vi "DAQ_FDV Meas Configure and Measure.vi"(0 "DAQmx Task In":refnum<k21>, 2 "Execution Settings":T1, 5 "Range and Terminal Settings":T6={"Global Settings"={"Min Range (V)"=-10.0, "Max Range (V)"=10.0, "Terminal Configuration"=10083}, "Specific Channel Settings"=[]} {"Specific Channel Settings"."Terminal Configuration" items=[""=0, "RSE"=10083, "NRSE"=10078, "Differential"=10106, "Pseudodifferential"=12529]; "Specific Channel Settings"."Max Range" format="%.2p"; "Specific Channel Settings"."Min Range" format="%.2p"; "Global Settings"."Terminal Configuration" items=["RSE"=10083, "NRSE"=10078, "Differential"=10106, "Pseudodifferential"=12529]; "Global Settings"."Max Range (V)" format="%.2p"; "Global Settings"."Min Range (V)" format="%.2p"}, 7 "Timing and Trigger Settings":T3={"Timing Settings"={"Sample Clock Source"="OnboardClock", "Sample Rate (Hz)"=10000.0, "Number of Samples"=1000, "Sample Timing Engine"=enum."Auto"}, "Trigger Settings"={"Trigger Type"=enum."No Trigger", "Digital Start Trigger Source"="", "Digital Start Trigger Edge"=10280}} {"Trigger Settings"."Digital Start Trigger Edge" items=["Rising"=10280, "Falling"=10171]; "Timing Settings"."Sample Rate (Hz)" format="%.2p"}, 11 "error in":errorcluster) -> (4 "DAQmx Task Out":refnum<k21>, 6 "Voltage Waveforms":waveform(dbl)[](graph), 8 "Frequency Domain Measurements":T8 {"Detected Tones"."Amplitudes (V)" format="%.2p"; "Detected Tones"."Frequencies (Hz)" format="%.2p"}, 10 "Acquisition Time (s)":dbl caption="Acq. Time Period (s)" format="%.2p", 15 "error out":errorcluster)   [LabVIEW 2021, in "DAQ_Frequency Domain Measurement.lvlib"]
doc: "Configure, initiate and fetch Frequency domain measurements from the channels configured."
uses:
  DAQ_Frequency Domain Measurement.lvlib
  Typedefs/Timing & Trigger Settings.ctl
  Typedefs/Timing Settings.ctl
  Signal Voltage Generation/Typedefs/Trigger Settings.ctl
  Typedefs/Range and Terminal Settings.ctl
  Typedefs/Specific Channel Settings.ctl
  Typedefs/FD Measurements.ctl
  Typedefs/Detected Tones.ctl
  Typedefs/Execution Settings.ctl
  Common/Typedefs/Execution Options - Measure.ctl
  <vilib>/DAQmx/read.llb/DAQmx Read (Analog 1D Wfm NChan NSamp).vi
  <vilib>/DAQmx/configure/timing.llb/DAQmx Timing (Sample Clock).vi
  <vilib>/DAQmx/configure/trigger.llb/DAQmx Start Trigger (Digital Edge).vi
  <vilib>/DAQmx/miscellaneous.llb/DAQmx Fill In Error Info.vi
  <resource>/objmgr/daqmx.rc
  Signal Voltage Generation/DAQ_Signal Voltage Generation.lvlib
panel:
  # "Inputs"
  # "Outputs"
  # "Min \nRange (V)"
  # "Max \nRange (V)"
  # "Terminal Configuration"
  # "Physical Channel Name"
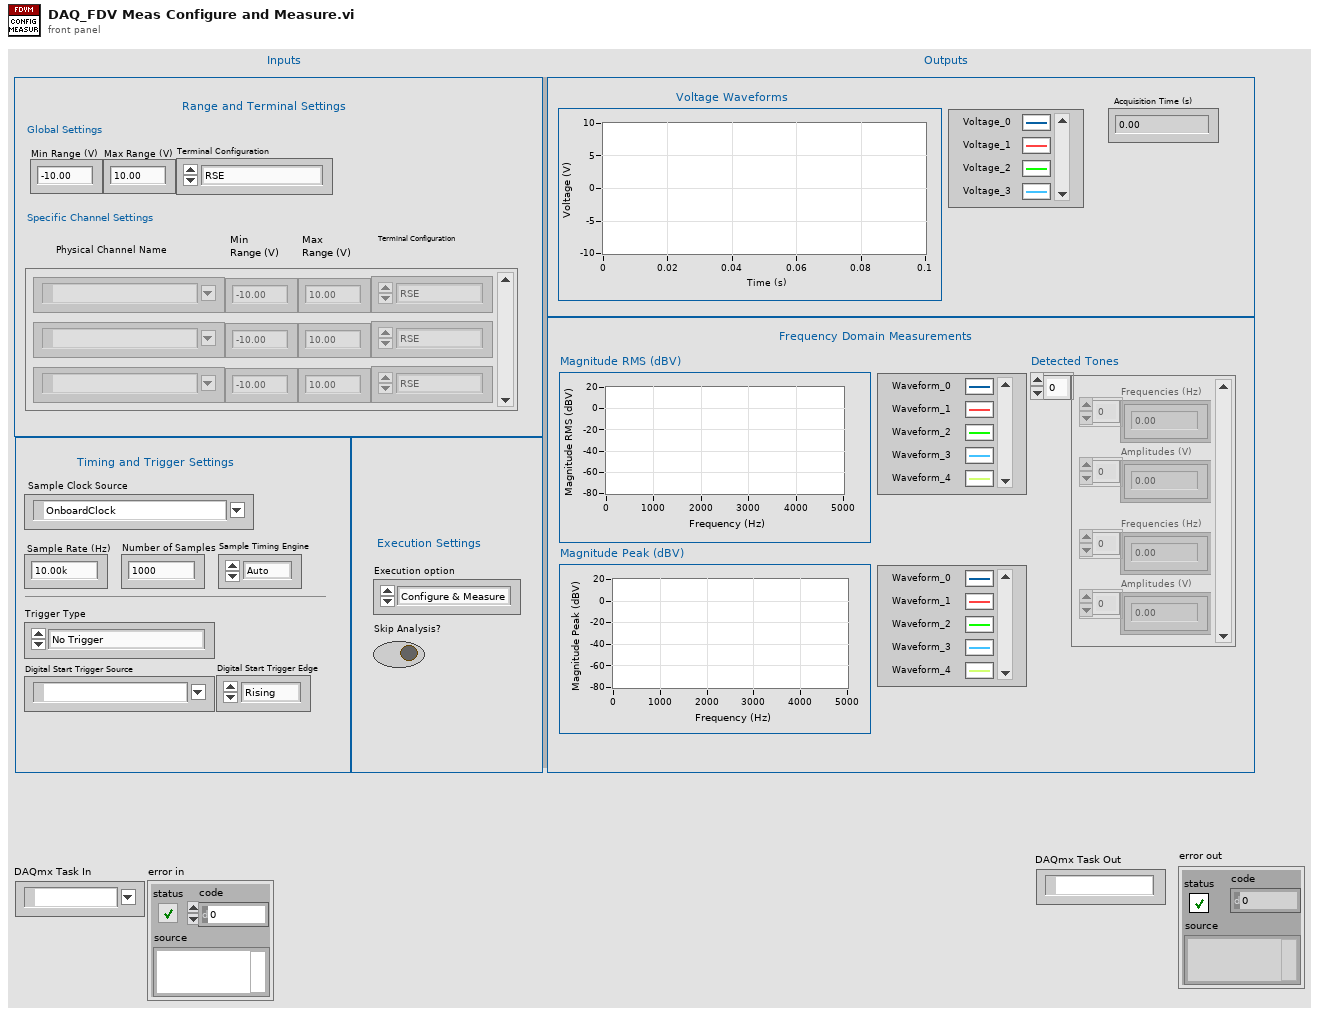
[diagram p1: front panel]
types:
  T1 = typedef "DAQ_Frequency Domain Measurement.lvlib/Execution Settings.ctl" = cluster{"Execution option":T2, "Skip Analysis?":bool}
  T2 = typedef "Execution Options - Measure.ctl" = enum16{"Configure & Measure", "Configure only", "Measure only"}
  T3 = typedef "DAQ_Frequency Domain Measurement.lvlib/Timing & Trigger Settings.ctl" = cluster{"Timing Settings":T4, "Trigger Settings":T5}
  T4 = typedef "DAQ_Frequency Domain Measurement.lvlib/Timing Settings.ctl" = cluster{"Sample Clock Source":tag, "Sample Rate (Hz)":dbl, "Number of Samples":i32, "Sample Timing Engine":enum16{"te0", "te1", "ai", "Auto"}}
  T5 = typedef "DAQ_Signal Voltage Generation.lvlib/Trigger Settings.ctl" = cluster{"Trigger Type":enum16{"No Trigger", "Digital Start"}, "Digital Start Trigger Source":tag, "Digital Start Trigger Edge":i32}
  T6 = typedef "DAQ_Frequency Domain Measurement.lvlib/Range and Terminal Settings.ctl" = cluster{"Global Settings":cluster{"Min Range (V)":dbl, "Max Range (V)":dbl, "Terminal Configuration":i32}, "Specific Channel Settings":T7[]}
  T7 = typedef "DAQ_Frequency Domain Measurement.lvlib/Specific Channel Settings.ctl" = cluster{"Active Channels":tag, "Min Range":dbl, "Max Range":dbl, "Terminal Configuration":i32}
  T8 = typedef "DAQ_Frequency Domain Measurement.lvlib/FD Measurements.ctl" = cluster{"Magnitude RMS (dBV)":cluster{"f0":dbl, "df":dbl, "magnitude":dbl[]}[], "Magnitude Peak (dBV)":cluster{"f0":dbl, "df":dbl, "magnitude":dbl[]}[], "Detected Tones":T9[]}
  T9 = typedef "DAQ_Frequency Domain Measurement.lvlib/Detected Tones.ctl" = cluster{"Frequencies (Hz)":dbl[], "Amplitudes (V)":dbl[]}
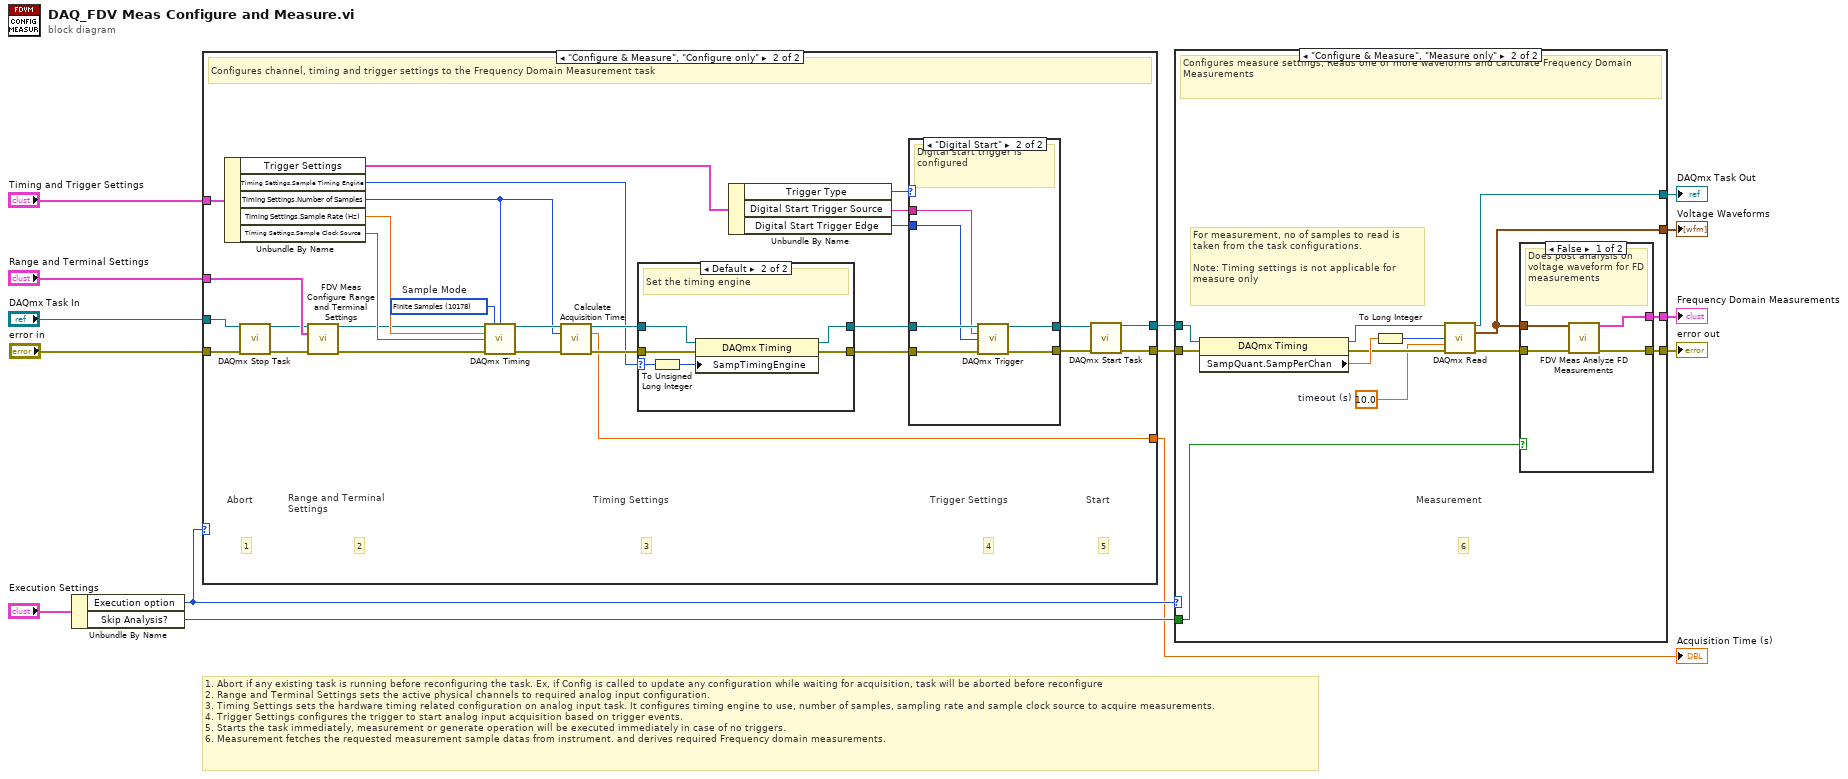
[diagram p0: block diagram]
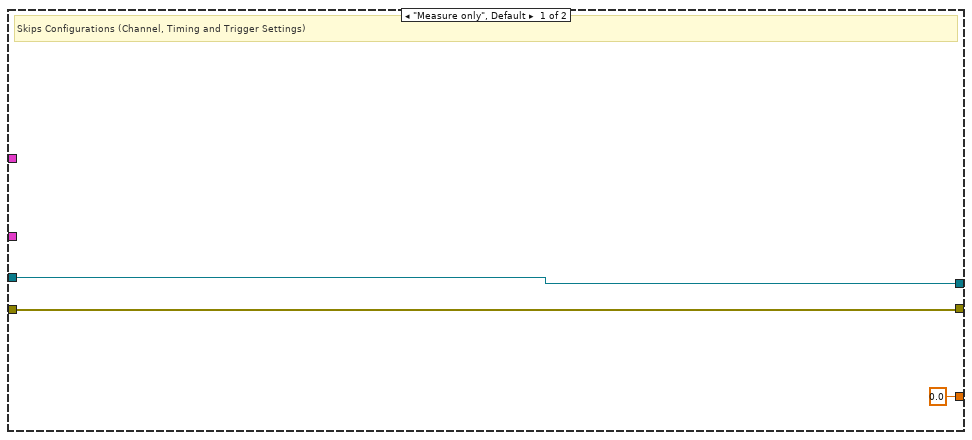
[diagram p2: hidden frame]
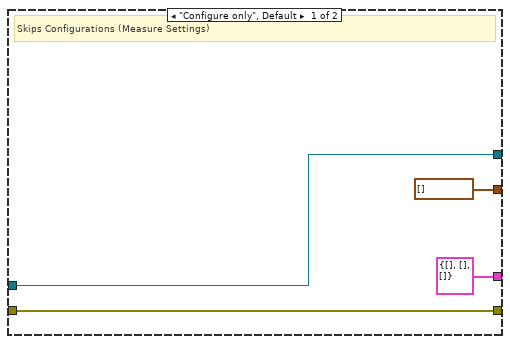
[diagram p5: hidden frame]
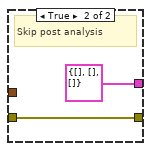
[diagram p6: hidden frame]
diagram:
  # "1. Abort if any existing task is running before reconfiguring the task. Ex, if Config is called to update any configuration while waiting for acquisition, task will be aborted before reconfigure\n2. Range and Terminal Settings sets the active physical channels to required analog input configuration.\n3. Timing Settings sets the hardware timing related configuration on analog input task. It configures timing engine to use, number of samples, sampling rate and sample clock source to acquire measurements.\n4. Trigger Settings configures the trigger to start analog input acquisition based on trigger events.\n5. Starts the task immediately, measurement or generate operation will be executed immediately in case of no triggers.\n6. Measurement fetches the requested measurement sample datas from instrument. and derives required Frequency domain measurements."
  n1 = Unbundle By Name("Execution Settings") -> ("Execution option"=w4:T2, "Skip Analysis?"=w3:bool)
  n2 = case shown="\"Configure & Measure\", \"Configure only\"" w4 {
    tunnel: "error in" -> [w17 w19]
    tunnel: "DAQmx Task In" -> [w16 w21]
    tunnel: "Timing and Trigger Settings" -> [_ w39]
    tunnel: [w16 w31] -> w13
    tunnel: [w17 w33] -> w14
    tunnel: "Range and Terminal Settings" -> [_ w24]
    tunnel: [0.0 ("Acquisition Time Period (s)") w18] -> w1
    frame "Measure only", Default {
      # "Skips Configurations (Channel, Timing and Trigger Settings)"
    }
    frame "Configure & Measure", "Configure only" {
      w43 = 10178 items=["Finite Samples"=10178, "Continuous Samples"=10123, "Hardware Timed Single Point"=12522]  # Sample Mode
      # "1"
      # "Abort"
      # "5"
      # "Start"
      # "4"
      # "3"
      # "2"
      # "Range and Terminal \nSettings"
      # "Trigger Settings"
      # "Timing Settings"
      # "Configures channel, timing and trigger settings to the Frequency Domain Measurement task"
      n3 = Unbundle By Name(w39) -> ("Trigger Settings"=w23:T5, "Timing Settings.Sample Timing Engine"=w34:enum16{"te0", "te1", "ai", "Auto"}, "Timing Settings.Number of Samples"=w30:i32, "Timing Settings.Sample Rate (Hz)"=w40:dbl, "Timing Settings.Sample Clock Source"=w41:tag)
      n4 = call <vilib>:"DAQmx Stop Task.vi"("task/channels in"=w21, "error in"=w19) -> ("task out"=w22:refnum<k21>, "error out"=w20:errorcluster)  [unwired: 12 in]
      n5 = call "FDV Meas Configure Range and Terminal Settings.vi"("DAQmx Task In"=w22, "Range and Terminal Settings"=w24, "error in (no error)"=w20) -> ("DAQmx Task Out"=w25:refnum<k21>, "error out"=w26:errorcluster)  [unwired: 11 in]
      n6 = call-poly <vilib>:"DAQmx Timing.vi"("task/channels in"=w25, "sample mode"=w43, "samples per channel"=w30, "rate"=w40, "source"=w41, "error in"=w26) -> ("task out"=w45:refnum<k21>, "error out"=w44:errorcluster)  [unwired: 8 in]
      n7 = call "Calculate Acquisition Time.vi"("Refnum in"=w45, "Number of Samples"=w30, "error in (no error)"=w44) -> ("Refnum out"=w36:refnum<k21>, "Acquisition Time Period (s)"=w18:dbl, "error out"=w42:errorcluster)  [unwired: 10 in]
      n8 = case shown="Default" w34 {
        selector: w34 -> [_ w49]
        tunnel: w42 -> [w47 w53]
        tunnel: [w47 w52] -> w37
        tunnel: w36 -> [w46 w51]
        tunnel: [w46 w50] -> w35
        frame "Auto" {
          # "Timing engine is auto-selected"
        }
        frame Default {
          # "Set the timing engine"
          n9 = To Unsigned Long Integer(number=w49) -> (unsigned 32bit integer=w48:u32)
          n10 = property class="DAQmx Timing"(reference=w51, error in=w53, "SampTimingEngine"=w48) -> (reference out=w50:refnum<k21>, error out=w52:errorcluster)
        }
      }
      n11 = Unbundle By Name(w23) -> ("Trigger Type"=w27:enum16{"No Trigger", "Digital Start"}, "Digital Start Trigger Source"=w29:tag, "Digital Start Trigger Edge"=w28:i32)
      n12 = case shown="\"Digital Start\"" w27 {
        tunnel: w35 -> [w55 w61]
        tunnel: w37 -> [w54 w60]
        tunnel: [w55 w59] -> w32
        tunnel: [w54 w58] -> w38
        tunnel: w29 -> [_ w57]
        tunnel: w28 -> [_ w56]
        frame "No Trigger", Default {
          # "No Trigger settings has been configured"
        }
        frame "Digital Start" {
          # "Digital start trigger is configured"
          n13 = call-poly <vilib>:"DAQmx Trigger.vi"("task/channels in"=w61, "source"=w57, "edge"=w56, "error in"=w60) -> ("task out"=w59:refnum<k21>, "error out"=w58:errorcluster)  [unwired: 10 in]
        }
      }
      n14 = call <vilib>:"DAQmx Start Task.vi"("task/channels in"=w32, "error in"=w38) -> ("task out"=w31:refnum<k21>, "error out"=w33:errorcluster)  [unwired: 12 in]
    }
  }
  "Acquisition Time (s)" <- w1
  n15 = case shown="\"Configure & Measure\", \"Measure only\"" w4 {
    tunnel: w13 -> [w65 w74]
    tunnel: w14 -> [w64 w71]
    tunnel: [w65 w76] -> w12
    tunnel: [w64 w78] -> w10
    tunnel: [T8 {"Magnitude RMS (dBV)"=[], "Magnitude Peak (dBV)"=[], "Detected Tones"=[]} ("Frequency Domain Measurements") w69] -> w6
    tunnel: w3 -> [_ w67]
    tunnel: [waveform(dbl)[] [] ("data") w66] -> w2
    frame "Configure only", Default {
      # "Skips Configurations (Measure Settings)"
    }
    frame "Configure & Measure", "Measure only" {
      w68 = 10.0  # timeout (s)
      # "For measurement, no of samples to read is taken from the task configurations.\n\nNote: Timing settings is not applicable for measure only"
      # "6"
      # "Measurement"
      # "Configures measure settings, Reads one or more waveforms and calculate Frequency Domain Measurements"
      n16 = property class="DAQmx Timing"(reference=w74, error in=w71) -> (reference out=w75:refnum<k21>, error out=w72:errorcluster, "SampQuant.SampPerChan"=w73:dbl)
      n17 = To Long Integer(number=w73) -> (32bit integer=w70:i32)
      n18 = call-poly <vilib>:"DAQmx Read.vi"("task/channels in"=w75, "number of samples per channel"=w70, "timeout"=w68, "error in"=w72) -> ("task out"=w76:refnum<k21>, "data"=w66:waveform(dbl)[], "error out"=w77:errorcluster)  [unwired: 9 in]
      n19 = case shown="False" w67 {
        tunnel: w66 -> [w82 _]
        tunnel: [w81 w84] -> w78
        tunnel: w77 -> [w80 w84]
        tunnel: [w79 T8 {"Magnitude RMS (dBV)"=[], "Magnitude Peak (dBV)"=[], "Detected Tones"=[]} ("Frequency Domain Measurements")] -> w69
        frame False {
          # "Does post analysis on voltage waveform for FD measurements"
          n20 = call "FDV Meas Analyze FD Measurements.vi"("Voltage Waveforms"=w82, "error in (no error)"=w80) -> ("Frequency Domain Measurements"=w79:T8, "error out"=w81:errorcluster)  [unwired: 12 in]
        }
        frame True {
          # "Skip post analysis"
        }
      }
    }
  }
  "error out" <- w10
  "DAQmx Task Out" <- w12
  "Frequency Domain Measurements" <- w6
  "Voltage Waveforms" <- w2
